vi "Swerve Drive Calculations.vi"(4 "Wheel Base Width":dbl=23.0, 5 "Wheel Base Length":dbl=20.0, 7 "Longitudinal - Y":dbl, 8 "Rotational - Z":dbl, 9 "Lateral - X":dbl) -> (0 "Back Right Drive":cluster{"Speed":dbl, "Angle":dbl}, 1 "Back Left Drive":cluster{"Speed":dbl, "Angle":dbl}, 2 "Front Right Drive":cluster{"Speed":dbl, "Angle":dbl}, 3 "Front Left  Drive":cluster{"Speed":dbl, "Angle":dbl})   [LabVIEW 2020]
panel:
  out "Cos(Alpha)":dbl
  out "Sin(Alpha)":dbl
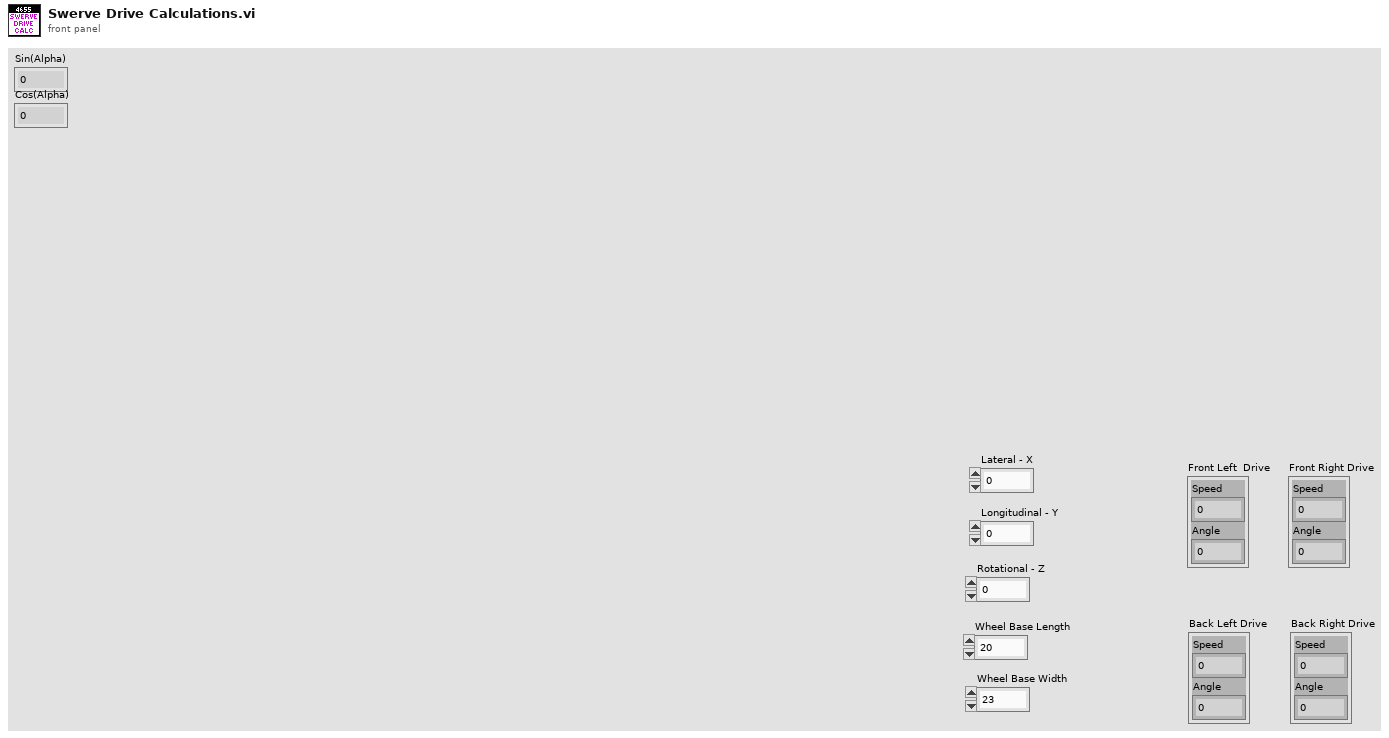
[diagram p1: front panel]
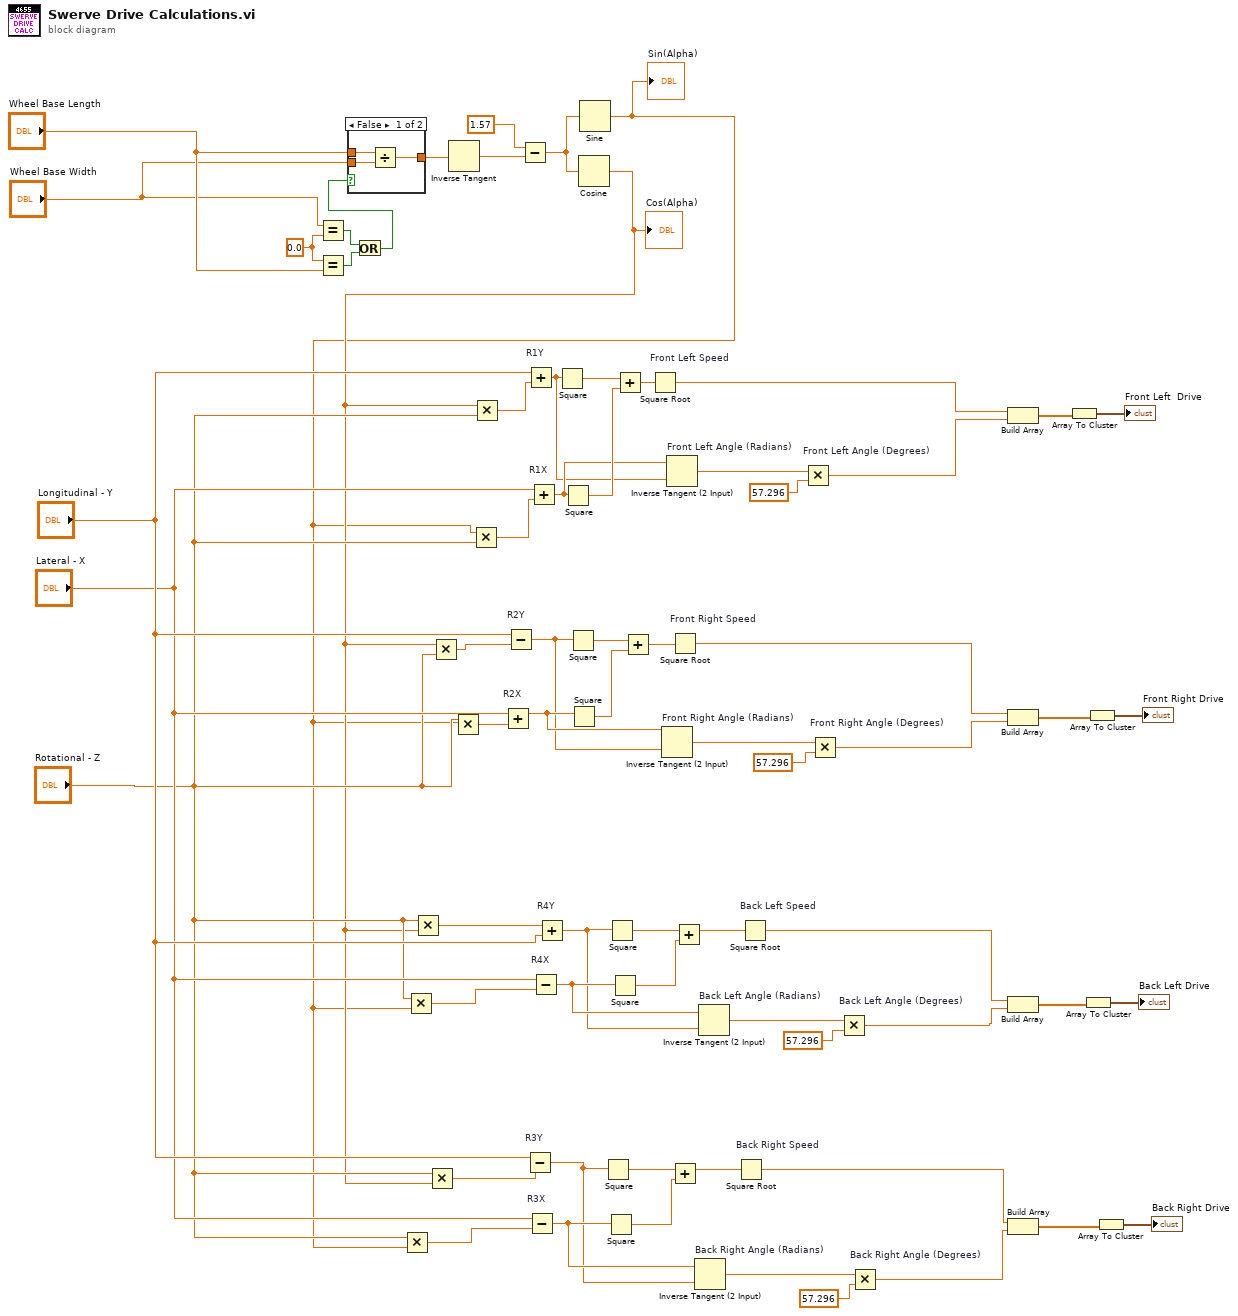
[diagram p0: block diagram]
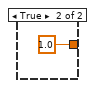
[diagram p2: hidden frame]
diagram:
  w9 = 0.0 ("y")
  n1 = Equal?(x="Wheel Base Width", y=w9) -> (x = y?=w8:bool)
  n2 = Equal?(x=w9, y="Wheel Base Length") -> (x = y?=w7:bool)
  n3 = Or(x=w8, y=w7) -> (x .or. y?=w5:bool)
  n4 = case shown="False" w5 {
    tunnel: [w70 1.0] -> w6
    tunnel: "Wheel Base Width" -> [w69 _]
    tunnel: "Wheel Base Length" -> [w68 _]
    frame False {
      n5 = Divide(x=w68, y=w69) -> (x/y=w70:dbl)
    }
    frame True {
    }
  }
  n6 = Inverse Tangent(1:w6) -> (0:w10:dbl)
  n7 = Subtract(x=1.57, y=w10) -> (x-y=w11:dbl)
  n8 = Cosine(x=w11) -> (cos(x)=w4:dbl)
  "Cos(Alpha)" <- w4
  n9 = Multiply(x="Rotational - Z", y=w4) -> (x*y=w49:dbl)
  n10 = Multiply(x="Rotational - Z", y=w4) -> (x*y=w32:dbl)
  n11 = Multiply(x=w4, y="Rotational - Z") -> (x*y=w58:dbl)
  n12 = Multiply(x=w4, y="Rotational - Z") -> (x*y=w67:dbl)
  n13 = Subtract "R2Y"(x="Longitudinal - Y", y=w58) -> (x-y=w52:dbl)
  n14 = Subtract "R3Y"(x="Longitudinal - Y", y=w32) -> (x-y=w35:dbl)
  n15 = Add "R1Y"(x="Longitudinal - Y", y=w67) -> (x+y=w61:dbl)
  n16 = Add "R4Y"(x=w49, y="Longitudinal - Y") -> (x+y=w43:dbl)
  n17 = Square(x=w61) -> (x^2=w63:dbl)
  n18 = Square(x=w52) -> (x^2=w56:dbl)
  n19 = Sine(x=w11) -> (sin(x)=w3:dbl)
  "Sin(Alpha)" <- w3
  n20 = Multiply(x="Rotational - Z", y=w3) -> (x*y=w40:dbl)
  n21 = Multiply(x="Rotational - Z", y=w3) -> (x*y=w48:dbl)
  n22 = Multiply(x="Rotational - Z", y=w3) -> (x*y=w57:dbl)
  n23 = Multiply(x=w3, y="Rotational - Z") -> (x*y=w66:dbl)
  n24 = Add "R2X"(x="Lateral - X", y=w57) -> (x+y=w53:dbl)
  n25 = Subtract "R3X"(x="Lateral - X", y=w40) -> (x-y=w36:dbl)
  n26 = Add "R1X"(x="Lateral - X", y=w66) -> (x+y=w62:dbl)
  n27 = Subtract "R4X"(x="Lateral - X", y=w48) -> (x-y=w44:dbl)
  n28 = Square(x=w62) -> (x^2=w65:dbl)
  n29 = Square(x=w53) -> (x^2=w55:dbl)
  n30 = Square(x=w35) -> (x^2=w39:dbl)
  n31 = Square(x=w36) -> (x^2=w38:dbl)
  n32 = Square(x=w43) -> (x^2=w47:dbl)
  n33 = Square(x=w44) -> (x^2=w46:dbl)
  n34 = Add(x=w63, y=w65) -> (x+y=w64:dbl)
  n35 = Add(x=w56, y=w55) -> (x+y=w54:dbl)
  n36 = Square Root "Front Left Speed"(x=w64) -> (sqrt(x)=w13:dbl)
  n37 = Inverse Tangent (2 Input) "Front Right Angle (Radians)"(1:w52, 2:w53) -> (0:w51:dbl)
  n38 = Inverse Tangent (2 Input) "Front Left Angle (Radians)"(1:w61, 2:w62) -> (0:w60:dbl)
  n39 = Square Root "Front Right Speed"(x=w54) -> (sqrt(x)=w19:dbl)
  n40 = Add(x=w39, y=w38) -> (x+y=w37:dbl)
  n41 = Add(x=w47, y=w46) -> (x+y=w45:dbl)
  n42 = Inverse Tangent (2 Input) "Back Right Angle (Radians)"(1:w35, 2:w36) -> (0:w34:dbl)
  n43 = Inverse Tangent (2 Input) "Back Left Angle (Radians)"(1:w43, 2:w44) -> (0:w42:dbl)
  n44 = Square Root "Back Right Speed"(x=w37) -> (sqrt(x)=w22:dbl)
  n45 = Square Root "Back Left Speed"(x=w45) -> (sqrt(x)=w18:dbl)
  n46 = Multiply "Front Left Angle (Degrees)"(x=w60, y=57.296) -> (x*y=w31:dbl)
  n47 = Multiply "Front Right Angle (Degrees)"(x=w51, y=57.296) -> (x*y=w20:dbl)
  n48 = Multiply "Back Left Angle (Degrees)"(x=w42, y=57.296) -> (x*y=w17:dbl)
  n49 = Multiply "Back Right Angle (Degrees)"(x=w34, y=57.296) -> (x*y=w21:dbl)
  n50 = Build Array(w13, w31) -> (w30:dbl[])
  n51 = Build Array(w19, w20) -> (w28:dbl[])
  n52 = Build Array(w18, w17) -> (w26:dbl[])
  n53 = Build Array(w22, w21) -> (w24:dbl[])
  n54 = Array To Cluster(array=w30) -> (cluster=→"Front Left  Drive":cluster{"[0]":dbl, "[1]":dbl})
  n55 = Array To Cluster(array=w26) -> (cluster=→"Back Left Drive":cluster{"[0]":dbl, "[1]":dbl})
  n56 = Array To Cluster(array=w28) -> (cluster=→"Front Right Drive":cluster{"[0]":dbl, "[1]":dbl})
  n57 = Array To Cluster(array=w24) -> (cluster=→"Back Right Drive":cluster{"[0]":dbl, "[1]":dbl})
